vi "SerialReadwithTimeout.vi"(4 "error in (no error)":errorcluster, 5 "Timeout Limit":dbl=10.0 format="%.2f", 6 "Bytes to Read":u32=1, 7 "Port Number":i32=1) -> (0 "error out":errorcluster, 1 "Timeout":bool=TRUE, 2 "Error Out":bool, 3 "Serial Read":string)   [LabVIEW 2019]
doc: "The Serial Read with Timeout VI will read the requested byte count unless a timeout condition is met first. The VI will wait a set amount of time for the requested bytes to become available at the serial port buffer. If the bytes do become available, the VI will read the characters and return immediately."
panel:
  # "PC:  0 = COM1, 1= COM2,...\nMac:  0 = Modem, 1 = Printer\nSun: 0 = ttya, 1 = ttyb,..."
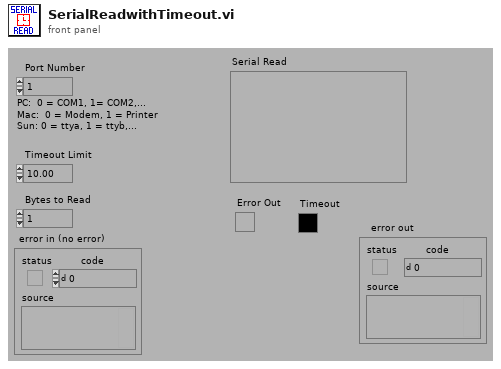
[diagram p1: front panel]
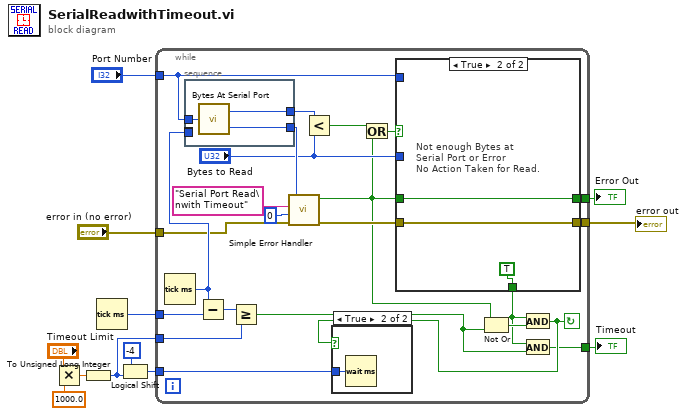
[diagram p0: block diagram]
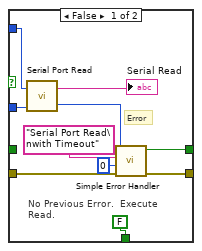
[diagram p3: hidden frame]
diagram:
  n1 = Multiply(x="Timeout Limit", y=1000.0) -> (x*y=w6:dbl)
  n2 = To Unsigned Long Integer(number=w6) -> (unsigned 32bit integer=w3:u32)
  n3 = Tick Count (ms)() -> (millisecond timer value=w11:u32)
  n4 = Logical Shift(y=i16 -4, x=w3) -> (x << y=w4:u32)
  n5 = while {
    tunnel: [w13] -> w1
    tunnel: "error in (no error)" -> [w14]
    tunnel: w3 -> [w17]
    tunnel: w4 -> [w19]
    tunnel: [w16] -> w9
    tunnel: [w31] -> w10
    tunnel: w11 -> [w35]
    tunnel: "Port Number" -> [w28]
    stop <- w18 continue-if-true
    n6 = Tick Count (ms)() -> (millisecond timer value=w20:u32)
    n7 = stacked-sequence {
      tunnel: w28 -> [w40]
      tunnel: [w39] -> w33
      tunnel: [w38] -> w34
      tunnel: [w37] -> _
      tunnel: w20 -> [w37]
      frame #0 {
        n8 = call <vilib>:"Bytes At Serial Port.vi"("port number"=w40) -> ("byte count"=w38:u32, "error code"=w39:i32)
      }
    }
    n9 = Subtract(x=w20, y=w35) -> (x-y=w23:u32)
    n10 = Greater Or Equal?(x=w23, y=w17) -> (x >= y?=w22:bool)
    n11 = call <vilib>:"Simple Error Handler.vi"("error code (no error:0)"=w33, "error source (\" \")"="Serial Port Read\nwith Timeout", "type of dialog (OK msg:1)"=0, "error in (no error)"=w14) -> ("error?"=w21:bool, "error out"=w27:errorcluster)  [unwired: 1 in, 3 out]
    n12 = Less?(x=w34, y="Bytes to Read") -> (x < y?=w29:bool)
    n13 = Or(x=w29, y=w21) -> (x .or. y?=w30:bool)
    n14 = case shown="True" w30 {
      tunnel: w28 -> [w46 _]
      tunnel: "Bytes to Read" -> [w50 _]
      tunnel: [w47 w53] -> w31
      tunnel: w21 -> [_ w53]
      tunnel: w27 -> [w45 w51]
      tunnel: [FALSE TRUE] -> w15
      tunnel: [w41 w51] -> w13
      frame False {
        # "No Previous Error.  Execute\nRead."
        # "Error"
        n15 = call <vilib>:"Serial Port Read.vi"("requested byte count"=w50, "port number"=w46) -> ("error code"=w48:i32, "string read"=→"Serial Read":string)
        n16 = call <vilib>:"Simple Error Handler.vi"("error code (no error:0)"=w48, "error source (\" \")"="Serial Port Read\nwith Timeout", "type of dialog (OK msg:1)"=0, "error in (no error)"=w45) -> ("error?"=w47:bool, "error out"=w41:errorcluster)  [unwired: 1 in, 3 out]
      }
      frame True {
        # "Not enough Bytes at\nSerial Port or Error\nNo Action Taken for Read."
      }
    }
    n17 = Not Or(1:w22, 2:w21) -> (0:w24:bool)
    n18 = And(x=w15, y=w24) -> (x .and. y?=w18:bool)
    n19 = case shown="True" w18 {
      tunnel: w19 -> [_ w36]
      frame False {
      }
      frame True {
        n20 = Wait (ms)(milliseconds to wait=w36) -> ()  [unwired: 1 out]
      }
    }
    n21 = And(x=w15, y=w22) -> (x .and. y?=w16:bool)
  }
  "Error Out" <- w10
  "Timeout" <- w9
  "error out" <- w1
